vi "Update Analog.vi"(8 "error in (no error)":errorcluster, 9 "Value":dbl, 10 "Channel Name":string, 11 "SoftVar Module in":refnum<class "SoftVar Module.lvclass">) -> (0 "error out":errorcluster, 3 "SoftVar Module out":refnum<class "SoftVar Module.lvclass">)   [LabVIEW 2020, in "Volatus.lvlib" / "SoftVar Module.lvclass"]
uses:
  SoftVar Module.lvclass
  SoftVar Module.lvclass/SoftVar Module.ctl
  lv-vecto/Vecto/Group/Group.lvclass
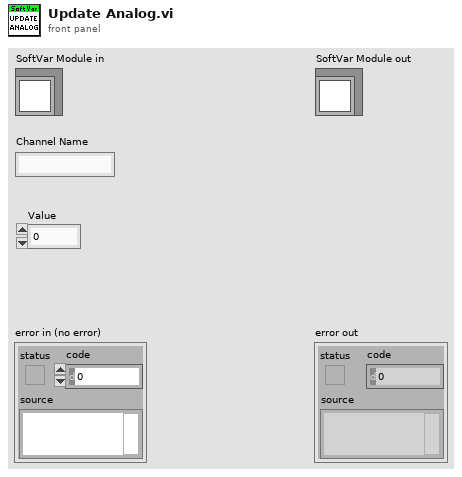
[diagram p1: front panel]
types:
  T1 = typedef "Volatus.lvlib/SoftVar Module.lvclass/Channel Info.ctl" = cluster{"Group Name":string, "Group Index":i32, "Index":i32}
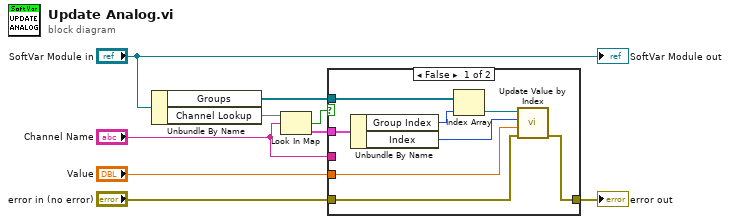
[diagram p0: block diagram]
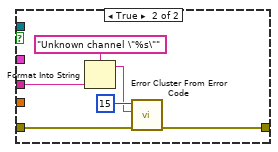
[diagram p2: hidden frame]
diagram:
  n1 = Unbundle By Name("SoftVar Module in") -> ("Groups"=w1:refnum<class "Group.lvclass">[], "Channel Lookup"=w8:map{string, T1})
  n2 = Look In Map(map=w8, key="Channel Name") -> (key not found?=w7:bool, value=w6:T1)  [unwired: 1 in]
  n3 = case shown="False" w7 {
    tunnel: w6 -> [w17 _]
    tunnel: "error in (no error)" -> [w11 w22]
    tunnel: "Value" -> [w12 _]
    tunnel: [w10 w21] -> w3
    tunnel: "Channel Name" -> [_ w20]
    tunnel: w1 -> [w16 _]
    frame False {
      n4 = Unbundle By Name(w17) -> ("Group Index"=w15:i32, "Index"=w13:i32)
      n5 = Index Array(array=w16, index=w15) -> (element=w14:refnum<class "Group.lvclass">)
      n6 = call "Update Value by Index.vi"("error in (no error)"=w11, "Scaled"=w12, "Index"=w13, "Group in"=w14) -> ("error out"=w10:errorcluster)  [unwired: 6 in, 1 out]
    }
    frame True {
      n7 = Format Into String(format string="Unknown channel \"%s\"", w20) -> (resulting string=w18:string)  [unwired: 2 in, 1 out]
      n8 = call <vilib>:"Error Cluster From Error Code.vi"("error in (no error)"=w22, "error message (\"\")"=w18, "error code (0)"=15) -> ("error out"=w21:errorcluster)  [unwired: 6 in]
    }
  }
  "error out" <- w3
  "SoftVar Module out" <- "SoftVar Module in"
